vi "GetXPos.vi"(7 "Menu":refnum<class "Menu.lvclass">, 9 "SubMenu":bool[](array[boolean]), 10 "Array":T1[](array[typedef]), 11 "Item Names":string[](array[string])) -> (1 "ShortCut Text":string[](array[string]), 2 "Start ShortCut":i16, 3 "Total X":i16)   [LabVIEW 2021, in "Menu.lvlib" / "Menu.lvclass"]
uses:
  Menu.lvclass
  Menu.lvclass/Menu.ctl
  Picture2D/src/Collection/Collection.lvclass
  Picture2D/src/Text/Text.lvclass
  Picture2D/src/PointSpecialized/PointSpecialized.lvclass
  Picture2D/src/2DPictureControl/2DPictureControl.lvclass
  Picture2D/src/Color/Color.lvclass
  Picture2D/src/Point/Point.lvclass
  C:/GitHub/Picture2D/src/Shape/Shape.lvclass
  C:/GitHub/Picture2D/src/Picture2D/Picture2D.lvclass
  C:/GitHub/Picture2D/src/IDrawable/IDrawable.lvclass
  C:/GitHub/Picture2D/src/IMovable/IMovable.lvclass
  C:/GitHub/Picture2D/src/IRotatable/IRotatable.lvclass
  C:/GitHub/Picture2D/src/IScalable/IScalable.lvclass
  C:/GitHub/Picture2D/src/Text/Text.lvclass
  C:/GitHub/Picture2D/src/Point/Point.lvclass
  C:/GitHub/Picture2D/src/PointSpecialized/PointSpecialized.lvclass
  C:/GitHub/Picture2D/src/Collection/Collection.lvclass
  <vilib>/Utility/miscctls.llb/LVMenuShortCut.ctl
panel:
  out "2D Picture out":picture
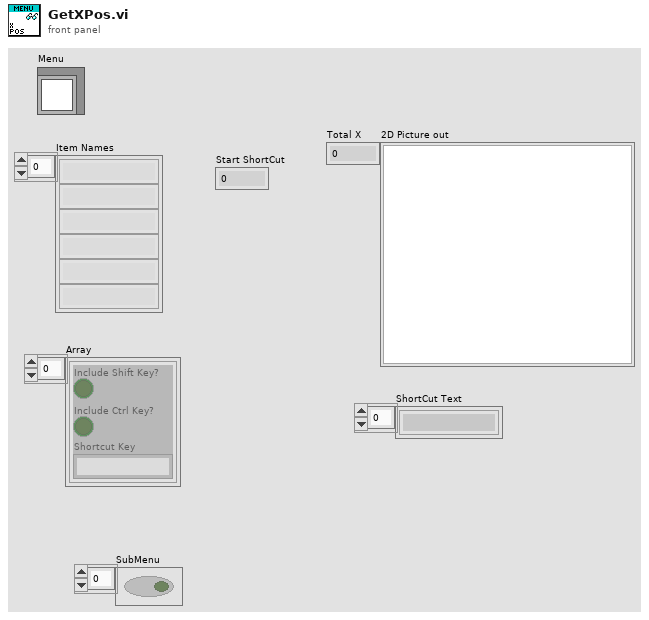
[diagram p1: front panel]
types:
  T1 = typedef "LVMenuShortCut.ctl" = cluster{"Include Shift Key?":bool, "Include Ctrl Key?":bool, "Shortcut Key":string}
  T2 = enum16{"User-specified Font", "Application Font", "System Font", "Dialog Font"}
  T3 = cluster{"left":i16, "top":i16, "right":i16, "bottom":i16}
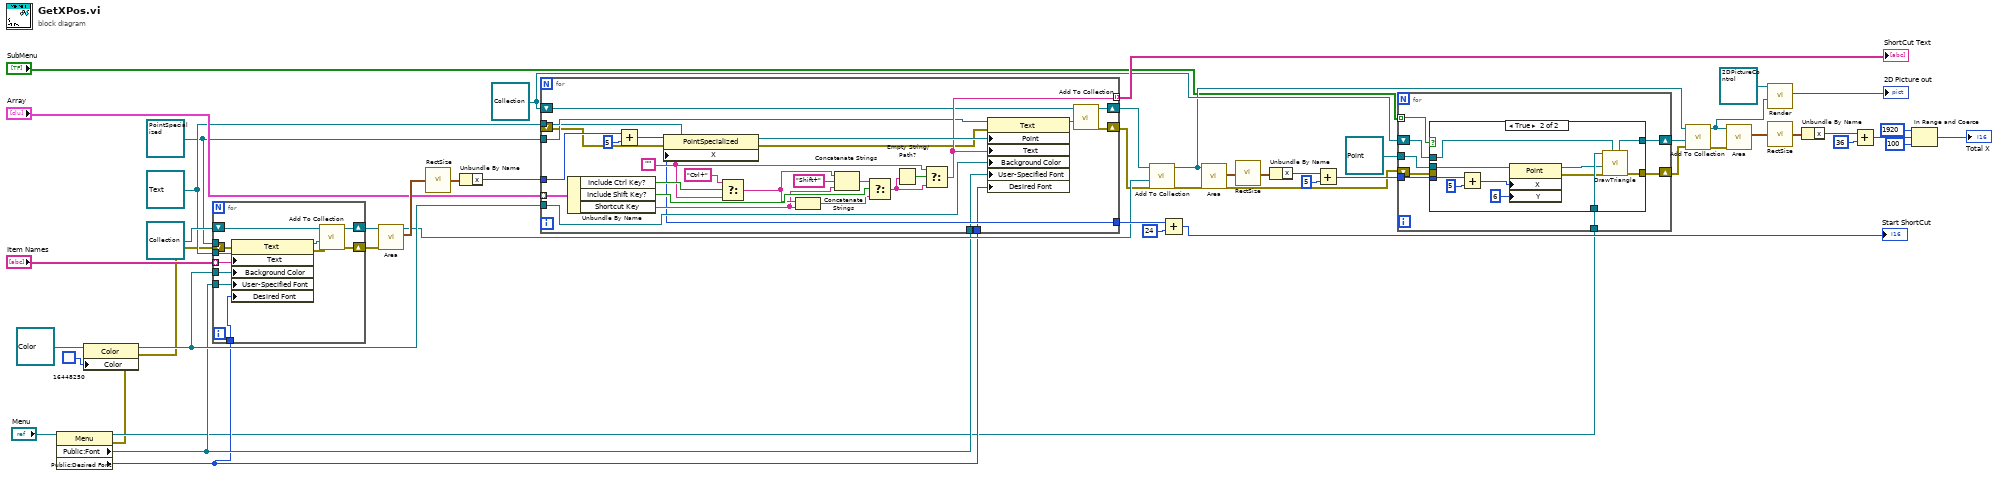
[diagram p0: block diagram]
diagram:
  w28 = refnum<class "Collection.lvclass"> refnum ("Picture2D.lvlib:Collection.lvclass")
  w36 = refnum<class "PointSpecialized.lvclass"> refnum ("Point")
  w37 = refnum<class "Text.lvclass"> refnum ("Text in")
  n1 = property class="Menu"(reference="Menu") -> (reference out=w9:refnum<class "Menu.lvclass">, error out=w2:errorcluster, "Public:Font"=w11:refnum<class "Font.lvclass">, "Public:Desired Font"=w10:T2)  [unwired: 1 in]
  n2 = property class="Color"(reference=refnum<class "Color.lvclass"> refnum ("Color"), error in=w2, "Color"=u32 16448250) -> (reference out=w35:refnum<class "Color.lvclass">, error out=w1:errorcluster)
  n3 = for {
    tunnel: w37 -> [w59]
    tunnel: "Item Names" -> [w60] mode=indexing
    shift-right: [w61] -> w49
    shift-left: refnum<class "Collection.lvclass"> refnum ("Picture2D.lvlib:Collection.lvclass") -> [w62]
    tunnel: w36 -> [_]
    tunnel: w35 -> [w57]
    tunnel: w11 -> [w56]
    tunnel: w10 -> [w55]
    shift-right: [w53] -> w3
    shift-left: w1 -> [w52]
    n4 = property class="Text"(reference=w59, error in=w52, "Text"=w60, "Background Color"=w57, "User-Specified Font"=w56, "Desired Font"=w55) -> (reference out=w58:refnum<class "Text.lvclass">, error out=w54:errorcluster)
    n5 = call-dynamic "Add To Collection.vi"("error in (no error)"=w54, "IDrawable"=w58, "Collection in"=w62) -> ("error out"=w53:errorcluster, "Collection out"=w61:refnum<class "Collection.lvclass">)  [unwired: 7 in]
  }
  n6 = call-dynamic "Area.vi"("error in (no error)"=w3, "Collection in"=w49) -> ("Area"=w50:T3, "Collection out"=w30:refnum<class "Collection.lvclass">)  [unwired: 7 in, 1 out]
  n7 = call <vilib>:"RectSize.vi"("rect"=w50) -> ("point"=w51:cluster{"x":i16, "y":i16})
  n8 = Unbundle By Name(w51) -> ("x"=w34:i16)
  n9 = for {
    tunnel: "Array" -> [w85] mode=indexing
    shift-right: [w82] -> w29
    shift-left: w28 -> [w68]
    tunnel: [w75] -> w39 mode=indexing
    tunnel: w37 -> [w74]
    tunnel: w36 -> [w73]
    tunnel: w34 -> [w72]
    tunnel: w35 -> [w71]
    tunnel: [w69] -> w33
    tunnel: w11 -> [w67]
    tunnel: w10 -> [w66]
    shift-right: [w65] -> w4
    shift-left: _ -> [w64]
    w80 = ""
    n10 = Unbundle By Name(w85) -> ("Include Ctrl Key?"=w89:bool, "Include Shift Key?"=w90:bool, "Shortcut Key"=w77:string)
    n11 = Add(x=w72, y=i16 5) -> (x+y=w69:i16)
    n12 = property class="PointSpecialized"(reference=w73, error in=w64, "X"=w69) -> (reference out=w83:refnum<class "PointSpecialized.lvclass">, error out=w63:errorcluster)
    n13 = Select(t="Ctrl+" ("f"), s=w89, f=w80) -> (s? t:f=w78:string)
    n14 = Concatenate Strings(w78, w77) -> (w76:string)
    n15 = Concatenate Strings(w78, "Shift+" ("f"), w77) -> (w86:string)
    n16 = Select(t=w86, s=w90, f=w76) -> (s? t:f=w79:string)
    n17 = Empty String/Path?(string/path=w79) -> (empty?=w81:bool)
    n18 = Select(t=w80, s=w81, f=w79) -> (s? t:f=w75:string)
    n19 = property class="Text"(reference=w74, error in=w63, "Point"=w83, "Text"=w75, "Background Color"=w71, "User-Specified Font"=w67, "Desired Font"=w66) -> (reference out=w84:refnum<class "Text.lvclass">)  [unwired: 1 out]
    n20 = call-dynamic "Add To Collection.vi"("IDrawable"=w84, "Collection in"=w68) -> ("error out"=w65:errorcluster, "Collection out"=w82:refnum<class "Collection.lvclass">)  [unwired: 8 in]
  }
  "ShortCut Text" <- w39
  n21 = call-dynamic "Add To Collection.vi"("error in (no error)"=w4, "IDrawable"=w30, "Collection in"=w29) -> ("error out"=w5:errorcluster, "Collection out"=w24:refnum<class "Collection.lvclass">)  [unwired: 7 in]
  n22 = Add(x=w33, y=i16 24) -> (x+y=→"Start ShortCut":i16)
  n23 = call-dynamic "Area.vi"("error in (no error)"=w5, "Collection in"=w24) -> ("error out"=w6:errorcluster, "Area"=w47:T3)  [unwired: 7 in, 1 out]
  n24 = call <vilib>:"RectSize.vi"("rect"=w47) -> ("point"=w46:cluster{"x":i16, "y":i16})
  n25 = Unbundle By Name(w46) -> ("x"=w41:i16)
  n26 = Add(x=w41, y=i16 5) -> (x+y=w26:i16)
  n27 = for {
    shift-right: [w98] -> w25
    shift-left: w28 -> [w97]
    tunnel: refnum<class "Point.lvclass"> refnum ("Point") -> [w96]
    tunnel: w26 -> [w95]
    tunnel: "SubMenu" -> [w94] mode=indexing
    tunnel: w9 -> [w93]
    shift-right: [w92] -> w8
    shift-left: w6 -> [w91]
    n28 = case shown="True" w94 {
      tunnel: [w100 w104] -> w98
      tunnel: w97 -> [w100 w105]
      tunnel: w96 -> [_ w111]
      tunnel: w95 -> [_ w110]
      tunnel: w93 -> [_ w106]
      tunnel: [w99 w101] -> w92
      tunnel: w91 -> [w99 _]
      frame False {
      }
      frame True {
        n29 = Add(x=w110, y=i16 5) -> (x+y=w109:i16)
        n30 = property class="Point"(reference=w111, "X"=w109, "Y"=i16 6 ("Point:y")) -> (reference out=w103:refnum<class "Point.lvclass">, error out=w102:errorcluster)  [unwired: 1 in]
        n31 = call "DrawTriangle.vi"("Collection in"=w105, "error in"=w102, "Point"=w103, "Menu in"=w106) -> ("error out"=w101:errorcluster, "Collection out"=w104:refnum<class "Collection.lvclass">)  [unwired: 5 in, 1 out]
      }
    }
  }
  n32 = call-dynamic "Add To Collection.vi"("error in (no error)"=w8, "IDrawable"=w25, "Collection in"=w24) -> ("error out"=w7:errorcluster, "Collection out"=w21:refnum<class "Collection.lvclass">)  [unwired: 7 in]
  n33 = call-dynamic "Area.vi"("error in (no error)"=w7, "Collection in"=w21) -> ("Area"=w19:T3)  [unwired: 7 in, 2 out]
  n34 = call-dynamic "Render.vi"("IDrawable"=w21, "2DPictureControl in"=refnum<class "2DPictureControl.lvclass"> refnum) -> ("2D Picture out"=→"2D Picture out":picture)  [unwired: 7 in, 2 out]
  n35 = call <vilib>:"RectSize.vi"("rect"=w19) -> ("point"=w20:cluster{"x":i16, "y":i16})
  n36 = Unbundle By Name(w20) -> ("x"=w18:i16)
  n37 = Add(x=w18, y=i16 36) -> (x+y=w17:i16)
  n38 = In Range and Coerce(upper limit=i16 1920, x=w17, lower limit=i16 100) -> (coerced(x)=→"Total X":i16)  [unwired: 1 out]
